vi "MPC-200 Wrapper for M command.vi"(8 "error in (no error)":errorcluster, 9 "Current Position":dbl[](array[numeric]), 10 "Move to Position":dbl[](array[numeric]), 11 "VISA resource name in":refnum<visa-resource-name>) -> (0 "error out":errorcluster, 3 "VISA resource name out":refnum<visa-resource-name>)   [LabVIEW 2015, in "XYZStage.lvlib"]
uses:
  XYZStage.lvlib
  <vilib>/Utility/error.llb/Error Cluster From Error Code.vi
  <vilib>/ErrorRing/Error Ring.xnode
panel:
  out "Delay (ms) for \"M\" cmd (0)":u32
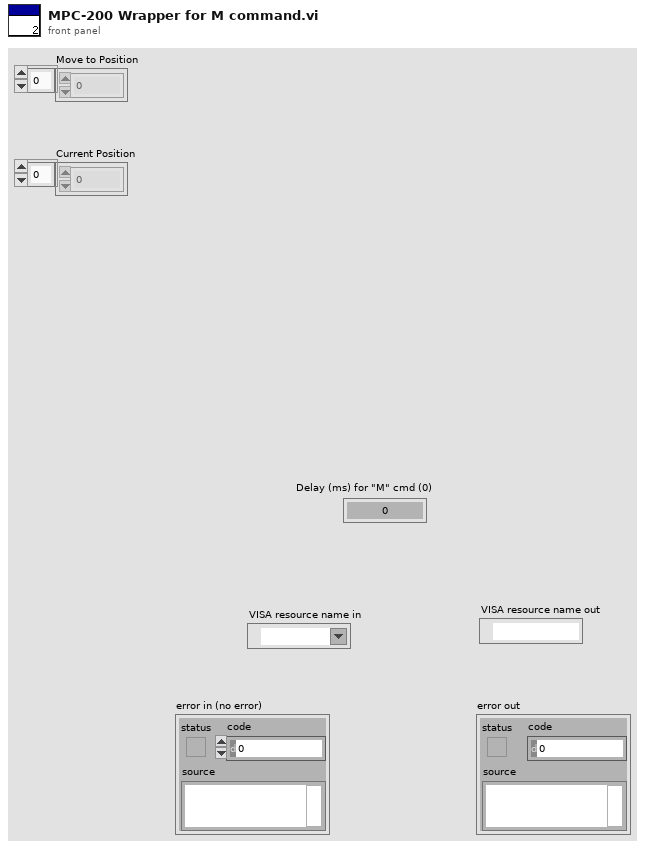
[diagram p1: front panel]
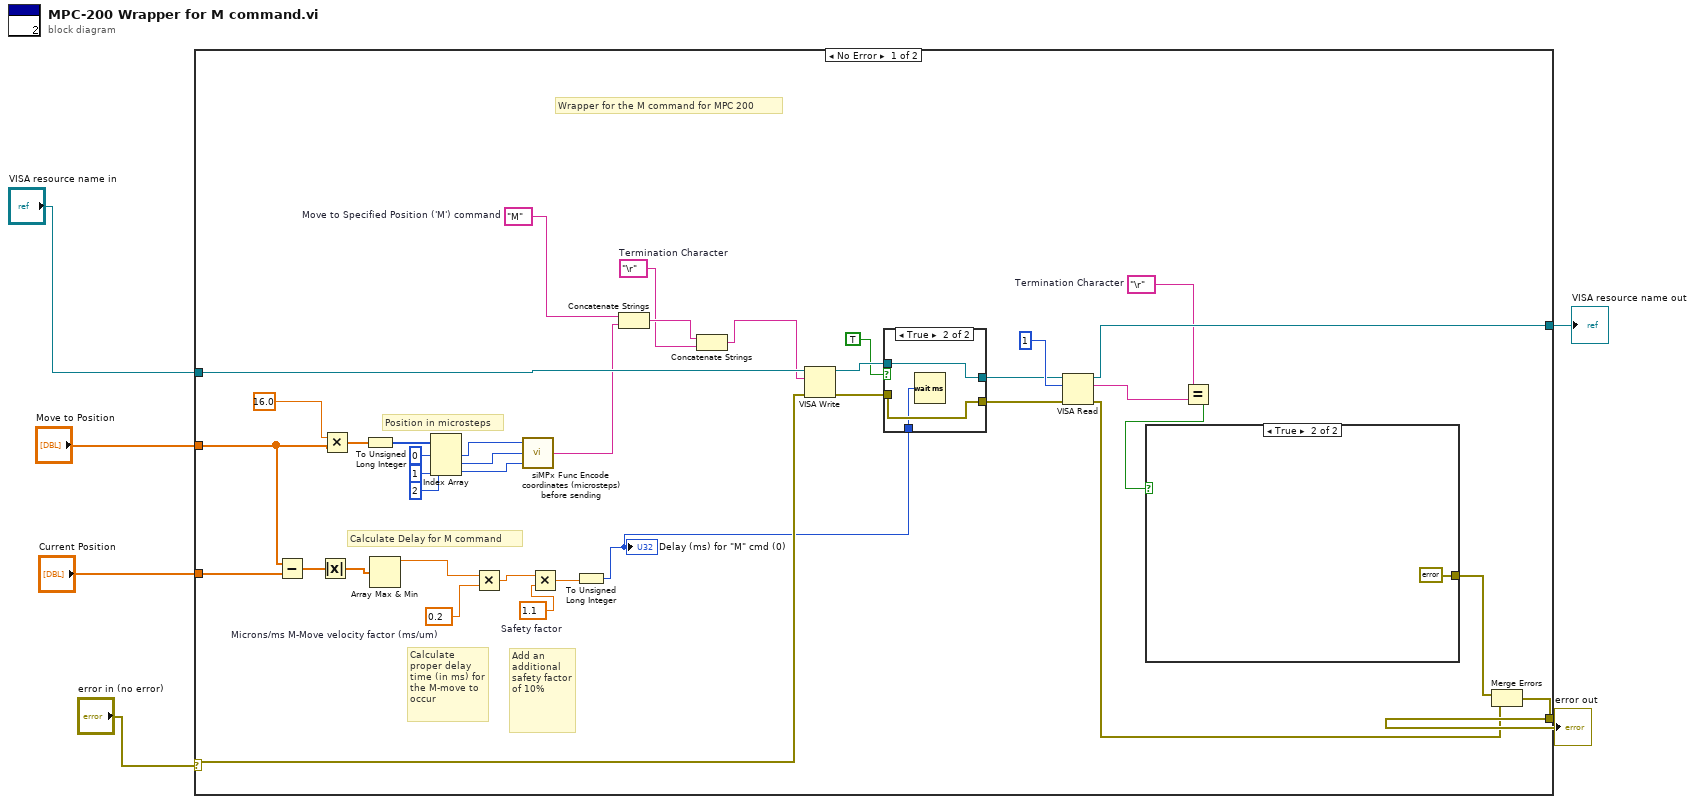
[diagram p0: block diagram]
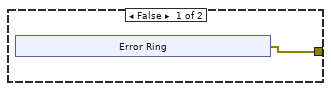
[diagram p2: hidden frame]
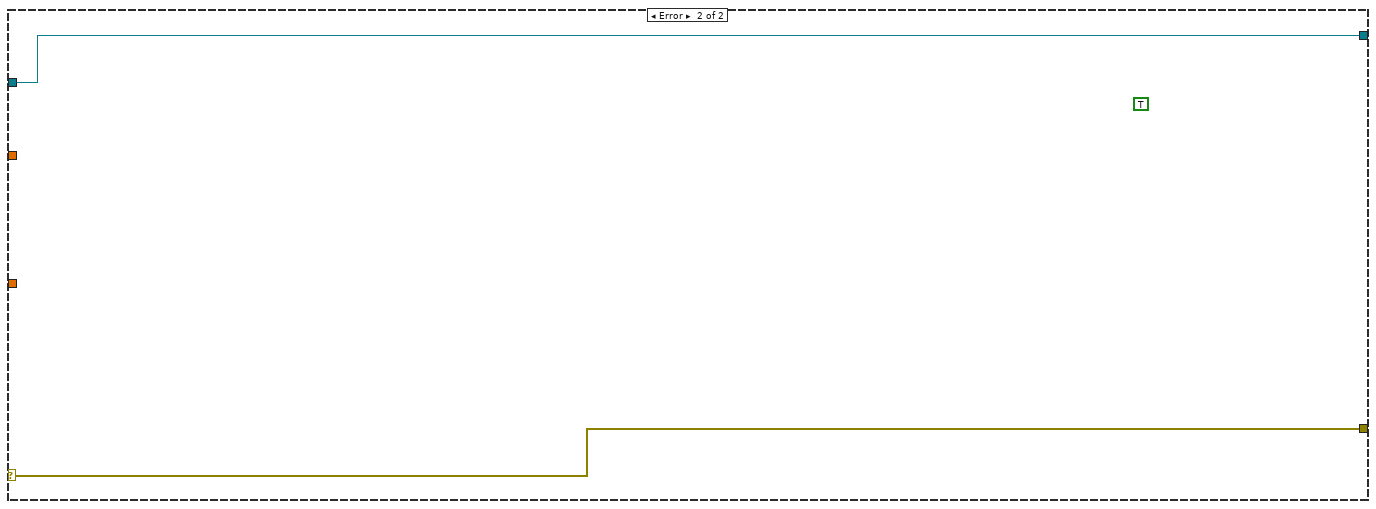
[diagram p4: hidden frame]
diagram:
  n1 = case shown="No Error" "error in (no error)" {
    selector: "error in (no error)" -> [w44 w59]
    tunnel: [w41 w59] -> w5
    tunnel: "VISA resource name in" -> [w45 w58]
    tunnel: [w42 w58] -> w3
    tunnel: "Move to Position" -> [w27 _]
    tunnel: "Current Position" -> [w28 _]
    frame No Error {
      w9 = "\r"  # Termination Character
      w11 = "\r"  # Termination Character
      w21 = 1.1  # Safety factor
      w23 = 0.2  # Microns/ms M-Move velocity factor (ms/um)
      w30 = "M"  # Move to Specified Position ('M') command
      # "Calculate Delay for M command"
      # "Add an additional safety factor of 10%"
      # "Calculate proper delay time (in ms) for the M-move to occur"
      # "Position in microsteps"
      # "Wrapper for the M command for MPC 200"
      n2 = Subtract(x=w27, y=w28) -> (x-y=w26:dbl[])
      n3 = Absolute Value(x=w26) -> (abs(x)=w25:dbl[])
      n4 = Multiply(x=16.0, y=w27) -> (x*y=w38:dbl[])
      n5 = To Unsigned Long Integer(number=w38) -> (unsigned 32bit integer=w37:u32[])
      n6 = Array Max & Min(array=w25) -> (max value=w24:dbl)  [unwired: 3 out]
      n7 = Index Array(array=w37, index #1=0 ("index"), index #2=1 ("index"), index #3=2 ("index")) -> (element #1=w33:u32, element #2=w32:u32, element #3=w31:u32)
      n8 = Multiply(x=w24, y=w23) -> (x*y=w22:dbl)
      n9 = call "siMPx Func Encode coordinates (microsteps) before sending.vi"("Z microsteps"=w31, "Y microsteps"=w32, "X microsteps"=w33) -> ("Coordinates string ready to send"=w29:string)
      n10 = Multiply(x=w22, y=w21) -> (x*y=w20:dbl)
      n11 = To Unsigned Long Integer(number=w20) -> (unsigned 32bit integer=w14:u32)
      "Delay (ms) for \"M\" cmd (0)" <- w14
      n12 = Concatenate Strings ("Concatenate strings into one command sequence")(w30, w29) -> (w13:string)
      n13 = Concatenate Strings(w13, w11) -> (w12:string)
      n14 = VISA Write(VISA resource name=w45, write buffer=w12, error in (no error)=w44) -> (VISA resource name out=w16:refnum<visa-resource-name>, error out=w18:errorcluster)  [unwired: 1 out]
      n15 = case shown="True" TRUE {
        tunnel: [w53 w57] -> w19
        tunnel: w18 -> [w53 w57]
        tunnel: [w54 w56] -> w17
        tunnel: w16 -> [w54 w56]
        tunnel: w14 -> [_ w55]
        frame False {
        }
        frame True {
          n16 = Wait (ms)(milliseconds to wait=w55) -> ()  [unwired: 1 out]
        }
      }
      n17 = VISA Read(VISA resource name=w17, byte count=u32 1, error in (no error)=w19) -> (VISA resource name out=w42:refnum<visa-resource-name>, read buffer=w10:string, error out=w40:errorcluster)  [unwired: 1 out]
      n18 = Equal?(x=w9, y=w10) -> (x = y?=w8:bool)
      n19 = case shown="True" w8 {
        tunnel: [w46 errorcluster {"status"=FALSE, "code"=0, "source"=""} ("error out")] -> w7
        frame False {
          n20 = xnode "Error Ring"() -> ("error out"=w46:errorcluster)
        }
        frame True {
        }
      }
      n21 = Merge Errors(w7, w40) -> (w41:errorcluster)
    }
    frame Error {
      (unwired) TRUE
    }
  }
  "VISA resource name out" <- w3
  "error out" <- w5
